vi "Matrix_NormF.vi"(11 "input matrix":T1) -> (0 "Error":bool, 3 "normF":dbl format="%.4f")   [LabVIEW 2019, in "Trajectory_Library.lvlib"]
doc: "Computes the Frobenius normal of the matrix.\n\n normF = Sqrt{ sum; i=1: m sum; j=1:n ( a[i,j] ^2 ) )\n\nInputs:\n - input matrix -- The input matrix\n\nOutputs:\n - NormF -- Double containing the frobenius normal value of this matrix\n - Error -- If TRUE, an error occured."
uses:
  <vilib>/Analysis/Matrix/Datatypes/RealMatrix.ctl
  Trajectory_Library.lvlib
  <vilib>/Analysis/NI_AALPro.lvlib
  <vilib>/Analysis/_algsub.llb/Real Matrix Norm.vi
  <vilib>/Analysis/Matrix/NI_Matrix.lvlib
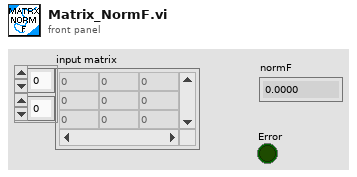
[diagram p1: front panel]
types:
  T1 = typedef "NI_Matrix.lvlib/RealMatrix.ctl" = dbl[][]
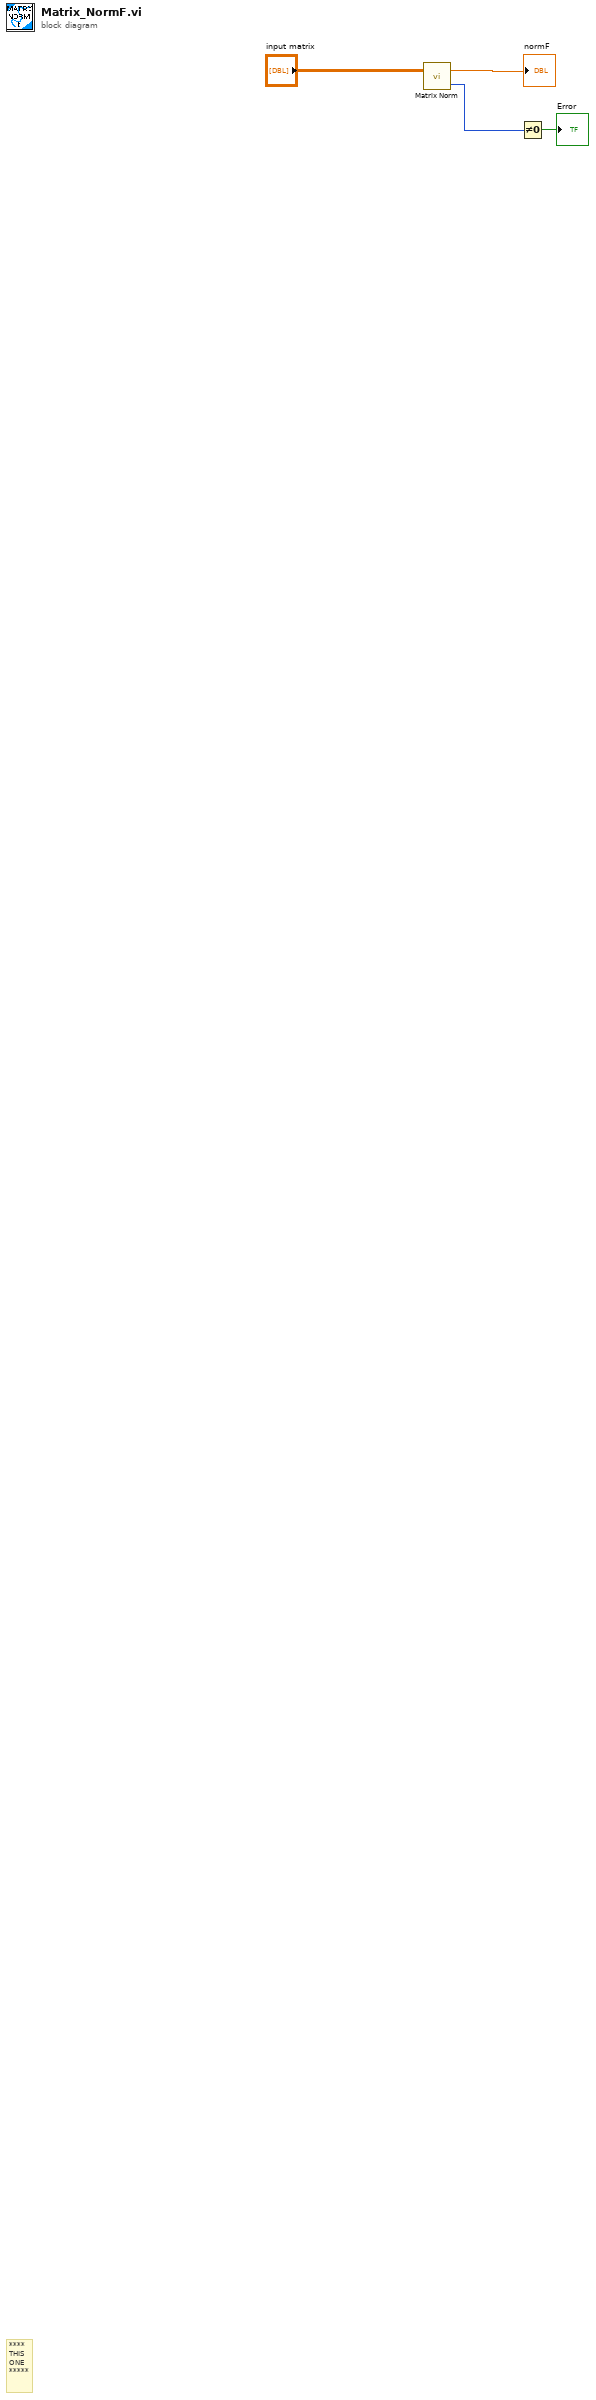
[diagram p0: block diagram]
diagram:
  # "****\nTHIS\nONE\n*****"
  n1 = call-poly <vilib>:"Matrix Norm.vi"("Input Matrix"="input matrix") -> ("error"=w3:i32, "norm"=→"normF":dbl)  [unwired: 1 in]
  n2 = Not Equal To 0?(x=w3) -> (x != 0?=→"Error":bool)
